vi "main.vi"() -> ()   [LabVIEW 2014]
uses:
  <vilib>/Utility/error.llb/Error Cluster From Error Code.vi
  <vilib>/ErrorRing/Error Ring.xnode
  Queue/Queue.lvlib
  <userlib>/NIST/NISTErrorLib/NISTErrorLib.lvlib
panel:
  in  "Stop Button":bool
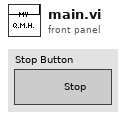
[diagram p1: front panel]
types:
  T1 = typedef "clUserEvents.ctl" = cluster{"StopEvent":refnum<user-event>}
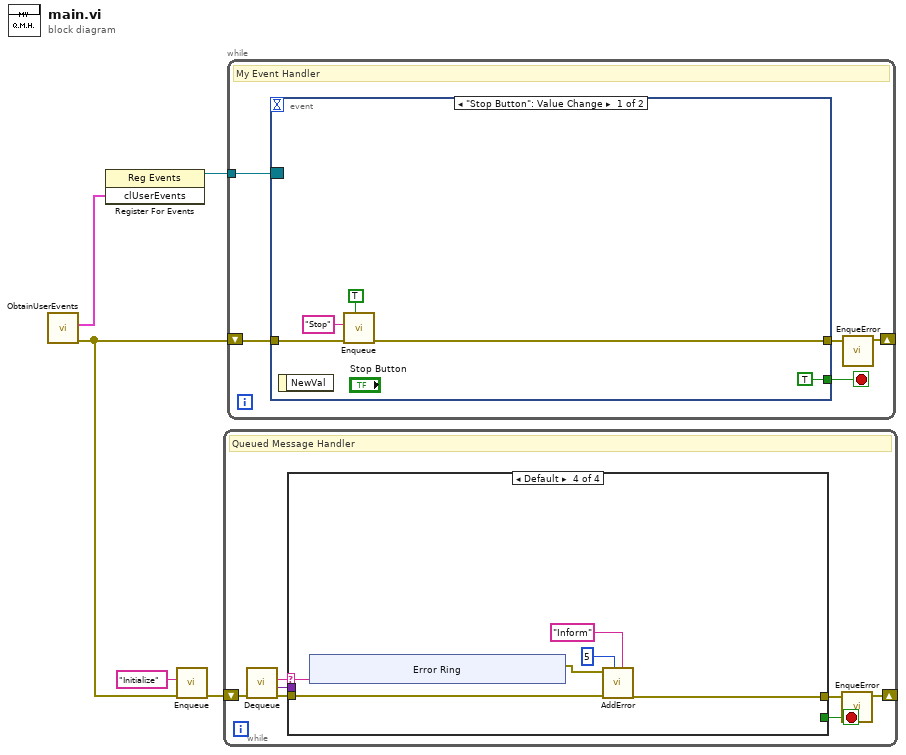
[diagram p0: block diagram]
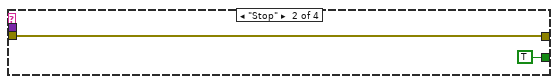
[diagram p3: hidden frame]
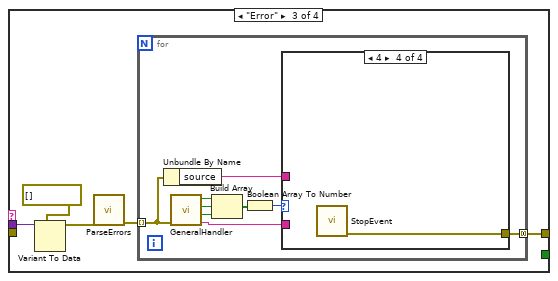
[diagram p4: hidden frame]
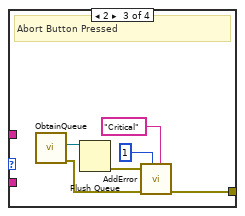
[diagram p8: hidden frame]
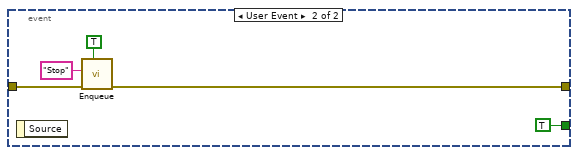
[diagram p9: hidden frame]
diagram:
  n1 = call "ObtainUserEvents.vi"() -> ("ErrorArray"=w3:errorcluster[], "clUserEvents"=w4:T1)  [unwired: 10 in]
  n2 = register-events(w4) -> (reference out=w5:refnum<event-registration>)  [unwired: 2 in, 1 out]
  n3 = call "Enqueue.vi"("ErrorArray"=w3, "Message"="Initialize") -> ("ErrorArray"=w1:errorcluster[])  [unwired: 9 in]
  n4 = while {
    shift-right: [w9] -> _
    shift-left: w1 -> [w12]
    stop <- w7 stop-if-true
    # "Queued Message Handler"
    n5 = call "Dequeue.vi"("ErrorArray"=w12) -> ("ErrorArray"=w8:errorcluster[], "Message Data"=w6:variant, "Message"=w11:string)  [unwired: 8 in]
    n6 = case shown="Default" w11 {
      selector: w11 -> [_ _ _ w43]
      tunnel: [w13 w15 w16 w41] -> w10
      tunnel: w8 -> [w13 w15 _ w40]
      tunnel: [_ TRUE _ _] -> w7
      tunnel: w6 -> [_ _ w20 _]
      frame "Initialize" {
      }
      frame "Stop" {
      }
      frame "Error" {
        n7 = Variant To Data(type=errorcluster[] [] ("ErrorArray"), Variant=w20) -> (data=w18:errorcluster[])  [unwired: 1 in, 1 out]
        n8 = call <userlib>:"ParseErrors.vi"("ErrorArray"=w18) -> ("ErrorArray"=w17:errorcluster[])  [unwired: 8 in, 2 out]
        n9 = for {
          tunnel: w17 -> [w29] mode=indexing
          tunnel: [w21] -> w16 mode=concatenating
          n10 = Unbundle By Name(w29) -> ("source"=w23:string)
          n11 = call <userlib>:"GeneralHandler.vi"("error in (no error)"=w29) -> ("Severity"=w22:string, "Stop"=w26:bool, "Abort"=w27:bool, "Continue"=w28:bool)  [unwired: 7 in]
          n12 = Build Array(w28, w27, w26) -> (w25:bool[])
          n13 = Boolean Array To Number(Boolean array=w25) -> (number=w24:u32)
          n14 = case shown="4" w24 {
            tunnel: w23 -> [_ _ _ _]
            tunnel: w22 -> [_ w30 _ _]
            tunnel: [_ _ w31 w37] -> w21
            frame 0, Default {
              # "No Dialog"
            }
            frame 1 {
              # "Continue"
              n15 = case shown="Default" w30 {
                frame Default {
                  # "Continue operation"
                }
                frame "Log" {
                  # "TODO: if your program\nhas a log file.  Write to \nit here."
                  # "Write to log file"
                }
              }
            }
            frame 2 {
              # "Abort Button Pressed"
              n16 = call "ObtainQueue.vi"() -> ("ErrorArray"=w34:errorcluster[], "QueueRef"=w36:refnum<queue>)  [unwired: 10 in]
              n17 = Flush Queue(queue=w36) -> (error out=w35:errorcluster)  [unwired: 1 in, 2 out]
              n18 = call <userlib>:"AddError.vi"("Severity"="Critical", "Priority"=u8 1, "ErrorArray"=w34, "error in (no error)"=w35) -> ("ErrorArray"=w31:errorcluster[])  [unwired: 6 in, 1 out]
            }
            frame 4 {
              n19 = call "StopEvent.vi"() -> ("ErrorArray"=w37:errorcluster[])  [unwired: 11 in]
            }
          }
        }
      }
      frame Default {
        n20 = xnode "Error Ring"("parameter 0"=w43) -> ("error out"=w42:errorcluster)
        n21 = call <userlib>:"AddError.vi"("Severity"="Inform", "Priority"=u8 5, "ErrorArray"=w40, "error in (no error)"=w42) -> ("ErrorArray"=w41:errorcluster[])  [unwired: 6 in, 1 out]
      }
    }
    n22 = call "EnqueError.vi"("ErrorArray"=w10) -> ("ErrorArray 2"=w9:errorcluster[])  [unwired: 10 in]
  }
  n23 = while {
    tunnel: w5 -> [w55]
    shift-right: [w52] -> _
    shift-left: w3 -> [w54]
    stop <- w51 stop-if-true
    # "My Event Handler"
    n24 = event shown="[0] \"Stop Button\": Value Change" {
      selector: w55 -> [_ _]
      dyn-events: _ -> [_ _]
      timeout: _ -> [_ _]
      tunnel: w54 -> [w60 w65]
      tunnel: [w59 w64] -> w53
      tunnel: [TRUE TRUE] -> w51
      event "Stop Button": Value Change {
        n25 = event-data() -> ()  [unwired: 1 in, 1 out]
        n26 = call "Enqueue.vi"("Priority (F)"=TRUE, "ErrorArray"=w60, "Message"="Stop") -> ("ErrorArray"=w59:errorcluster[])  [unwired: 8 in]
      }
      event User Event {
        n27 = event-data() -> ()  [unwired: 1 in, 1 out]
        n28 = call "Enqueue.vi"("Priority (F)"=TRUE, "ErrorArray"=w65, "Message"="Stop") -> ("ErrorArray"=w64:errorcluster[])  [unwired: 8 in]
      }
    }
    n29 = call "EnqueError.vi"("ErrorArray"=w53) -> ("ErrorArray 2"=w52:errorcluster[])  [unwired: 10 in]
  }
